vi "parse_AccelWithCovariance.vi"(4 "error in":errorcluster, 7 "msg in":string) -> (0 "error out":errorcluster, 2 "AccelCovariance":T1, 3 "msg out":string)   [LabVIEW 2012]
doc: "Parses a message into an acceleration with covariance"
uses:
  <userlib>/ROS for LabVIEW Software/ROS/MessageParsing/std_msgs/subs/parse_float64_array.vi
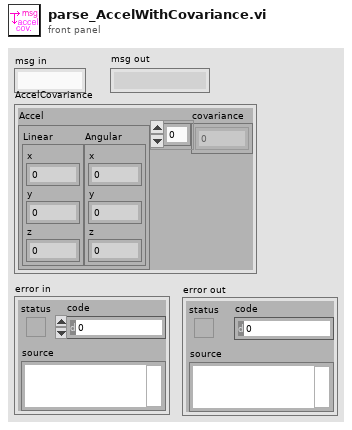
[diagram p1: front panel]
types:
  T1 = cluster{"Accel":cluster{"Linear":cluster{"x":dbl, "y":dbl, "z":dbl}, "Angular":cluster{"x":dbl, "y":dbl, "z":dbl}}, "covariance":dbl[]}
  T2 = cluster{"Linear":cluster{"x":dbl, "y":dbl, "z":dbl}, "Angular":cluster{"x":dbl, "y":dbl, "z":dbl}}
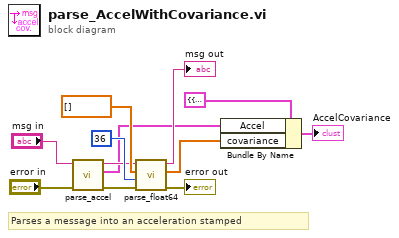
[diagram p0: block diagram]
diagram:
  # "Parses a message into an acceleration stamped"
  n1 = call "parse_accel.vi"("error in"="error in", "msg in"="msg in") -> ("error out"=w5:errorcluster, "Accel"=w3:T2, "msg out"=w6:string)  [unwired: 3 in]
  n2 = call-poly <userlib>:"parse_float64.vi"("error in"=w5, "Array Size"=36, "type"=dbl[] [], "msg in"=w6) -> ("error out"=→"error out":errorcluster, "number"=w2:dbl[], "msg out"=→"msg out":string)  [unwired: 1 in]
  n3 = Bundle By Name(cluster=T1 {"Accel"={"Linear"={"x"=0.0, "y"=0.0, "z"=0.0}, "Angular"={"x"=0.0, "y"=0.0, "z"=0.0}}, "covariance"=[]} ("AccelCovariance"), "Accel"=w3, "covariance"=w2) -> (→"AccelCovariance":T1)
